vi "Main - ESTF.vi"() -> ()   [LabVIEW 2015]
uses:
  Custom Controls/Main Menu.ctl
  <vilib>/DAQmx/read.llb/DAQmx Read (Analog 1D Wfm NChan NSamp).vi
  <vilib>/DAQmx/miscellaneous.llb/DAQmx Fill In Error Info.vi
  <vilib>/DAQmx/configure/task.llb/DAQmx Configure Logging (TDMS).vi
panel:
  out "Shot complete":bool
  out "Test Permit":bool
  out "HV Enable On?":bool
  in  "stop":bool
  out "HV On Relay":bool
  out "Earthed":bool
  out "Safety System Interlock":bool
  out "Menu":T1
  in  "Max Test Voltage (V)":dbl format="%#_4p"
  in  "Stick Type":string
  in  "Submit Setup":bool
  in  "Test Sequence":T2(array[cluster]) {"Total Test Energy (J)" format="%#_4p"}
  in  "Log File Folderpath":path
  out "Test Information":T3(array[cluster])
  in  "View last Summary":bool
  in  "Unlock Encloure Door":bool
  in  "Back to Setup 2":bool
  in  "Back to Setup":bool
  in  "Data Display":T4(tab)
  out "System Voltage":waveform(dbl)(graph)
  out "Measured Current":waveform(dbl)(graph)
  out "Measured Temperature":waveform(dbl)(graph)
  out "Measured PD Voltage":waveform(dbl)(graph)
  out "Elapsed Time (s)":dbl
  out "Cooldown time":dbl
  out "Pulses":i32
  out "Pulse No.":i32
  in  "Create Report":bool
  in  "Finish":bool
  in  "Show Log file":bool
  out "Total Test Energies":dbl[](array[numeric])
  # "Waiting for HV Enable Switch..."
  # "Waiting for Start Sequence button to be pressed..."
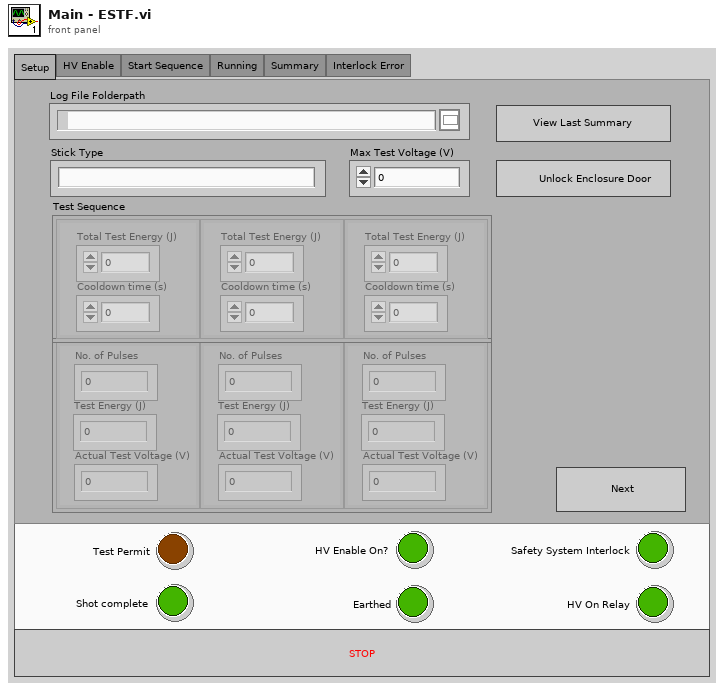
[diagram p1: front panel]
types:
  T1 = typedef "Main Menu.ctl" = enum32{"Setup", "HV Enable", "Start Sequence", "Running", "Summary", "Interlock Error"}
  T2 = cluster{"Cooldown time (s)":dbl, "Total Test Energy (J)":dbl}[]
  T3 = cluster{"No. of Pulses":i32, "Test Energy (J)":dbl, "Actual Test Voltage (V)":dbl}[]
  T4 = enum32{"Voltage", "Current", "Temperature", "PD Voltage"}
  T5 = cluster{"No. of Pulses":i32, "Test Energy (J)":dbl, "Actual Test Voltage (V)":dbl}
  T6 = enum16{"open", "open or create", "create or replace", "create", "open (read-only)"}
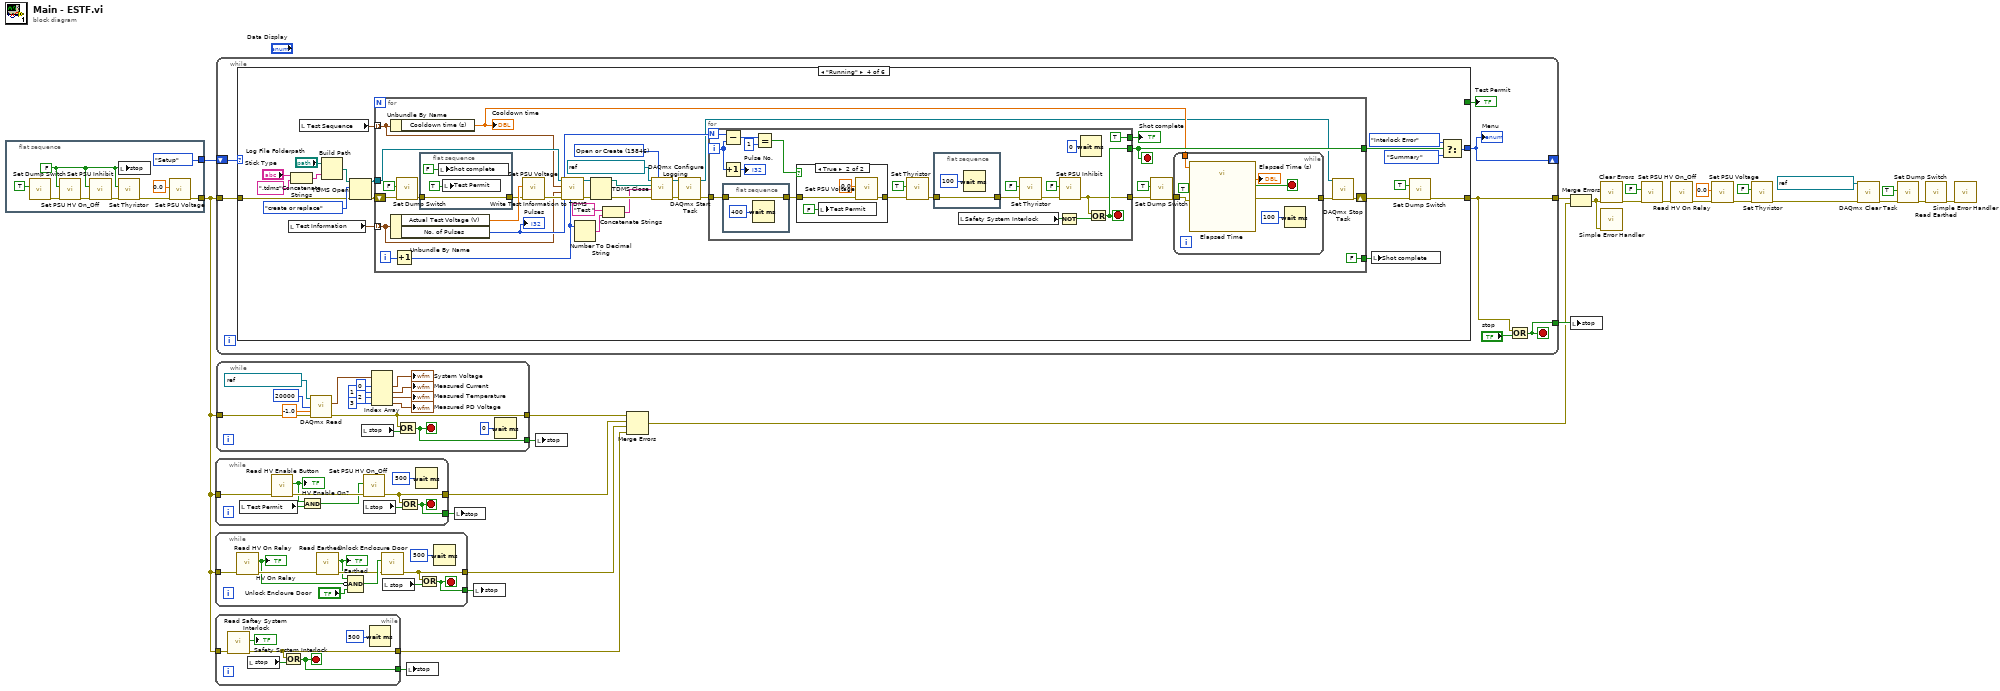
[diagram p0: block diagram]
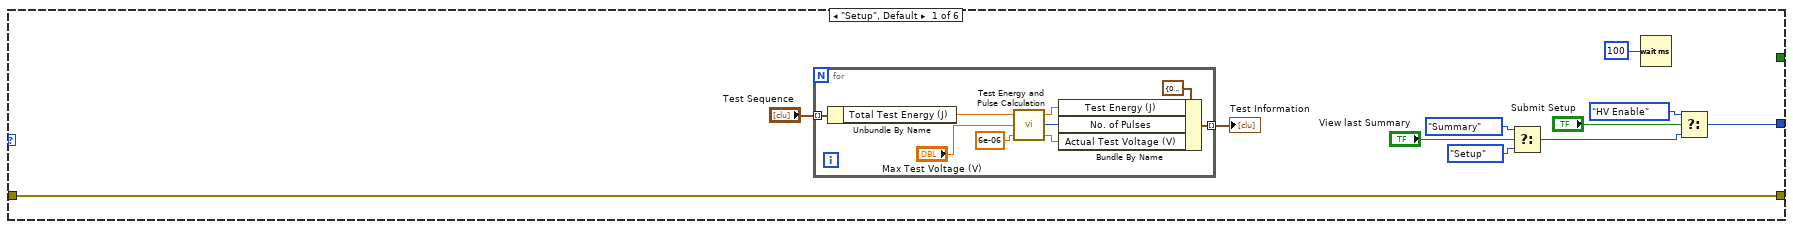
[diagram p2: hidden frame]
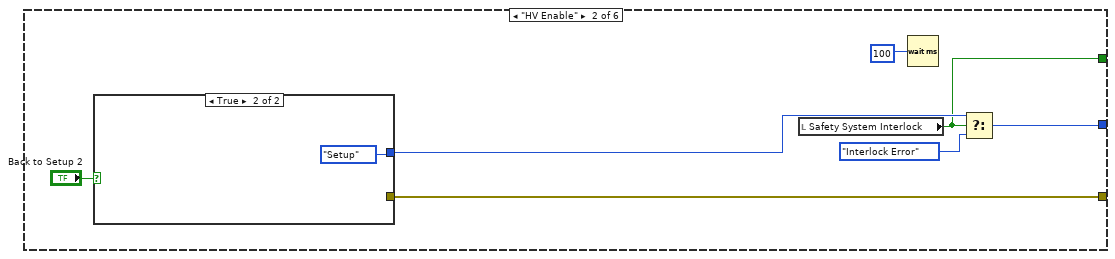
[diagram p3: hidden frame]
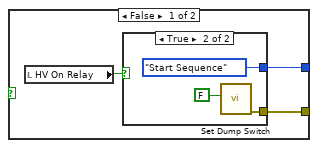
[diagram p4: hidden frame]
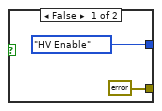
[diagram p5: hidden frame]
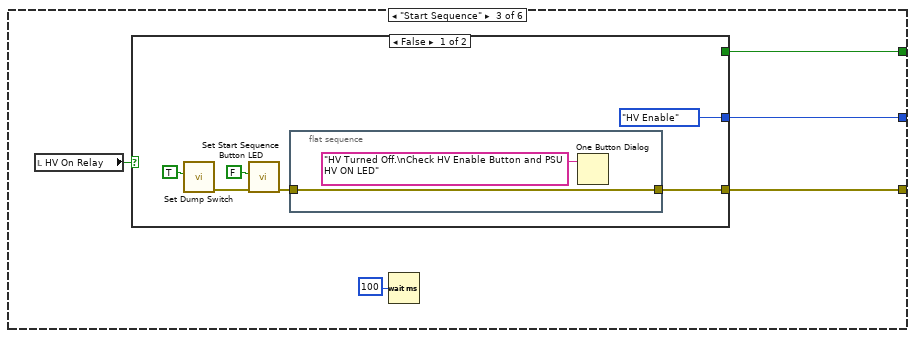
[diagram p6: hidden frame]
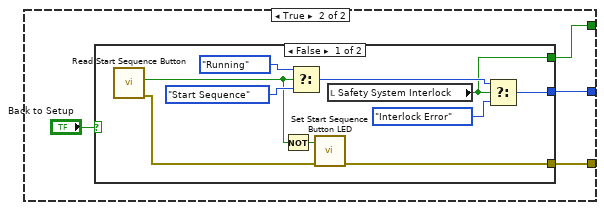
[diagram p7: hidden frame]
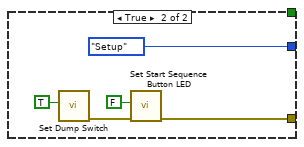
[diagram p8: hidden frame]
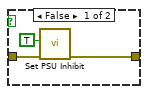
[diagram p9: hidden frame]
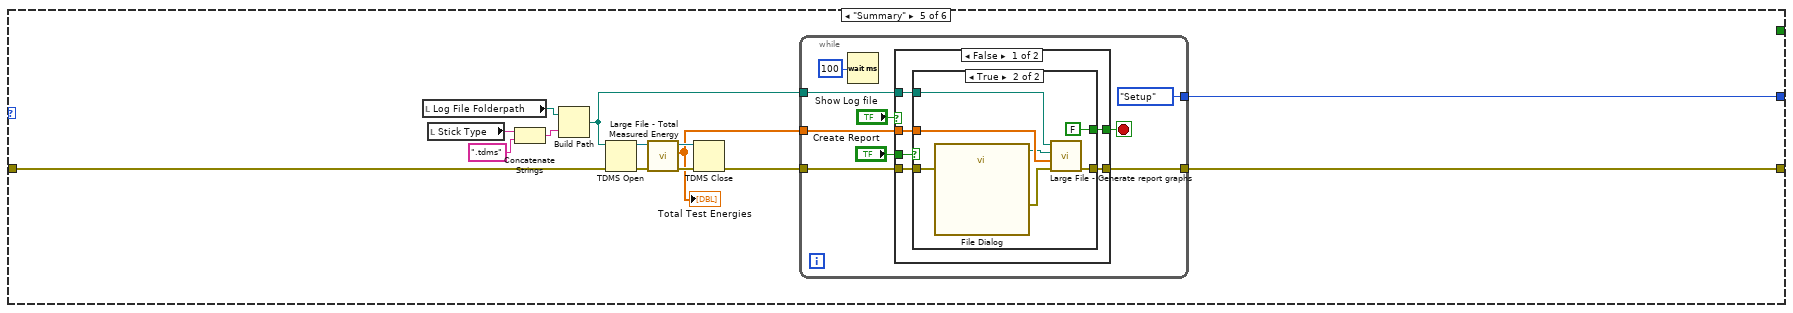
[diagram p10: hidden frame]
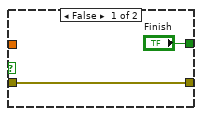
[diagram p11: hidden frame]
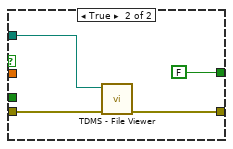
[diagram p12: hidden frame]
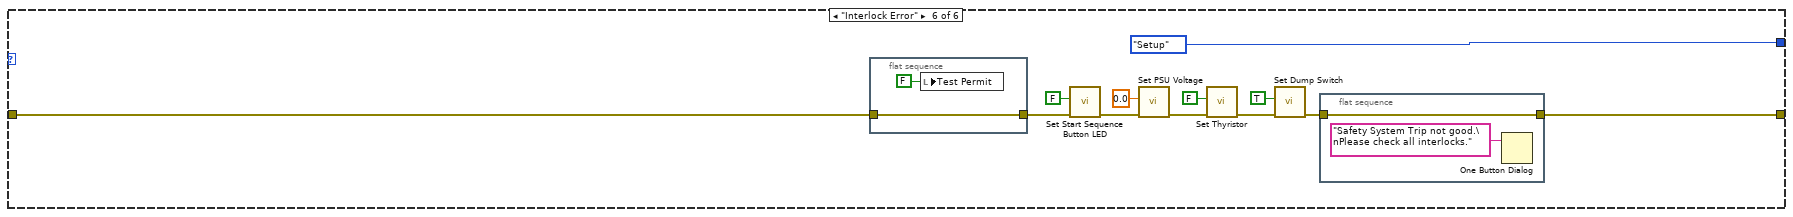
[diagram p13: hidden frame]
diagram:
  n1 = flat-sequence {
    tunnel: [Main_Menu."Setup" ("Menu")] -> w27
    tunnel: [w33] -> w4
    frame #0 {
      w28 = FALSE ("stop")
      n2 = call "Set Dump Switch.vi"("Earth"=TRUE) -> ("error out"=w32:errorcluster)  [unwired: 6 in]
      n3 = call "Set PSU HV On_Off.vi"("error in"=w32, "On/Off"=w28) -> ("error out"=w31:errorcluster)  [unwired: 5 in]
      n4 = call "Set PSU Inhibit.vi"("error in"=w31, "On/Off"=w28) -> ("error out"=w30:errorcluster)  [unwired: 5 in]
      n5 = call "Set Thyristor.vi"("error in"=w30, "On/Off"=w28) -> ("error out"=w29:errorcluster)  [unwired: 5 in]
      n6 = local write "stop"(w28) -> ()
      n7 = call "Set PSU Voltage.vi"("error in"=w29, "Voltage"=0.0) -> ("error out"=w33:errorcluster)  [unwired: 5 in]
    }
  }
  n8 = while {
    tunnel: [w40] -> w10
    tunnel: w4 -> [w39]
    tunnel: [w38] -> w7
    stop <- w40 stop-if-true
    n9 = local read "Test Permit"() -> (w42:bool)
    n10 = call "Read HV Enable Button.vi"("error in"=w39) -> ("error out"=w45:errorcluster, "HV Enable Pressed?"=w43:bool)  [unwired: 5 in]
    "HV Enable On?" <- w43
    n11 = And(x=w43, y=w42) -> (x .and. y?=w44:bool)
    n12 = call "Set PSU HV On_Off.vi"("error in"=w45, "On/Off"=w44) -> ("error out"=w38:errorcluster)  [unwired: 5 in]
    n13 = local read "stop"() -> (w41:bool)
    n14 = Or(x=w38, y=w41) -> (x .or. y?=w40:bool)
    n15 = Wait (ms)(milliseconds to wait=u32 500) -> ()  [unwired: 1 out]
  }
  n16 = while {
    tunnel: [w51] -> w11
    tunnel: w4 -> [w48]
    tunnel: [w47] -> w5
    stop <- w51 stop-if-true
    n17 = call "Read HV On Relay.vi"("error in"=w48) -> ("error out"=w56:errorcluster, "HV On Relay"=w55:bool)  [unwired: 5 in]
    "HV On Relay" <- w55
    n18 = call "Read Earthed.vi"("error in"=w56) -> ("error out"=w53:errorcluster, "Dump Switch mimic"=w50:bool)  [unwired: 5 in]
    "Earthed" <- w50
    n19 = Compound Arithmetic op=AND(w50, invert w55, "Unlock Encloure Door") -> (w54:bool)
    n20 = call "Unlock Enclosure Door.vi"("error in"=w53, "Unlock Encloure Door"=w54) -> ("error out"=w47:errorcluster)  [unwired: 5 in]
    n21 = local read "stop"() -> (w52:bool)
    n22 = Or(x=w47, y=w52) -> (x .or. y?=w51:bool)
    n23 = Wait (ms)(milliseconds to wait=u32 500) -> ()  [unwired: 1 out]
  }
  n24 = while {
    tunnel: [w61] -> w12
    tunnel: w4 -> [w59]
    tunnel: [w58] -> w6
    stop <- w61 stop-if-true
    n25 = call "Read Saftey System Interlock.vi"("error in"=w59) -> ("error out"=w58:errorcluster, "Safety System Interlock"=→"Safety System Interlock":bool)  [unwired: 5 in]
    n26 = local read "stop"() -> (w60:bool)
    n27 = Or(x=w58, y=w60) -> (x .or. y?=w61:bool)
    n28 = Wait (ms)(milliseconds to wait=u32 500) -> ()  [unwired: 1 out]
  }
  n29 = while {
    shift-right: [w66] -> _
    shift-left: w27 -> [w67]
    tunnel: [w68] -> w25
    tunnel: w4 -> [w64]
    tunnel: [w63] -> w1
    stop <- w68 stop-if-true
    n30 = case shown="\"Running\"" w67 {
      tunnel: [w75 w95 w110 w140 w246 Main_Menu."Setup" ("Menu")] -> w66
      tunnel: [w70 w92 w109 w138 w244 w278] -> w63
      tunnel: [_ w91 w108 _ _ _] -> w65
      tunnel: w64 -> [w70 _ _ w144 w243 w275]
      frame "Setup", Default {
        n31 = for {
          tunnel: "Test Sequence" -> [w87] mode=indexing
          tunnel: [w81] -> w78 mode=indexing
          n32 = Unbundle By Name(w87) -> ("Total Test Energy (J)"=w86:dbl)
          n33 = call "Test Energy and Pulse Calculation.vi"("Capacitor Size (f)"=6e-06, "Max Test Voltage (V)"="Max Test Voltage (V)", "Stick Energy (J)"=w86) -> ("Actual Test Voltage (V)"=w82:dbl, "Actual No. of Pulses"=w83:i32, "Actual Pulse Energy (J)"=w84:dbl)
          n34 = Bundle By Name(cluster=T5 {"No. of Pulses"=0, "Test Energy (J)"=0.0, "Actual Test Voltage (V)"=0.0} ("Test Information 2"), "Test Energy (J)"=w84, "No. of Pulses"=w83, "Actual Test Voltage (V)"=w82) -> (w81:T5)
        }
        "Test Information" <- w78
        n35 = Select(t=Main_Menu."Summary" ("Menu"), s="View last Summary", f=Main_Menu."Setup" ("Menu")) -> (s? t:f=w73:T1)
        n36 = Wait (ms)(milliseconds to wait=u32 100) -> ()  [unwired: 1 out]
        n37 = Select(t=Main_Menu."HV Enable" ("Menu"), s="Submit Setup", f=w73) -> (s? t:f=w75:T1)
      }
      frame "HV Enable" {
        n38 = case shown="True" "Back to Setup 2" {
          tunnel: [w99 Main_Menu."Setup" ("Menu")] -> w96
          tunnel: [w98 _] -> w92
          frame False {
            n39 = local read "HV On Relay"() -> (w97:bool)
            n40 = case shown="True" w97 {
              tunnel: [Main_Menu."HV Enable" ("Menu") Main_Menu."Start Sequence" ("Menu")] -> w99
              tunnel: [errorcluster {"status"=FALSE, "code"=0, "source"=""} ("error out") w102] -> w98
              frame False {
              }
              frame True {
                n41 = call "Set Dump Switch.vi"("Earth"=FALSE) -> ("error out"=w102:errorcluster)  [unwired: 6 in]
              }
            }
          }
          frame True {
          }
        }
        n42 = local read "Safety System Interlock"() -> (w91:bool)
        n43 = Wait (ms)(milliseconds to wait=u32 100) -> ()  [unwired: 1 out]
        n44 = Select(t=w96, s=w91, f=Main_Menu."Interlock Error" ("Menu")) -> (s? t:f=w95:T1)
      }
      frame "Start Sequence" {
        n45 = local read "HV On Relay"() -> (w106:bool)
        n46 = case shown="False" w106 {
          tunnel: [Main_Menu."HV Enable" ("Menu") w122] -> w110
          tunnel: [w112 w121] -> w109
          tunnel: [_ w120] -> w108
          frame False {
            n47 = call "Set Dump Switch.vi"("Earth"=TRUE) -> ("error out"=w113:errorcluster)  [unwired: 6 in]
            n48 = call "Set Start Sequence Button LED.vi"("error in"=w113, "Start LED"=FALSE) -> ("error out"=w111:errorcluster)  [unwired: 5 in]
            n49 = flat-sequence {
              tunnel: [w117] -> w112
              tunnel: w111 -> [w117]
              frame #0 {
                n50 = One Button Dialog(message="HV Turned Off.\nCheck HV Enable Button and PSU HV ON LED") -> ()  [unwired: 1 in, 1 out]
              }
            }
          }
          frame True {
            n51 = case shown="False" "Back to Setup" {
              tunnel: [w128 Main_Menu."Setup" ("Menu")] -> w122
              tunnel: [w127 w136] -> w121
              tunnel: [w125 _] -> w120
              frame False {
                n52 = call "Read Start Sequence Button.vi"() -> ("error out"=w123:errorcluster, "Start Button Pressed?"=w124:bool)  [unwired: 6 in]
                n53 = Not(x=w124) -> (.not. x?=w126:bool)
                n54 = Select(t=Main_Menu."Running" ("Menu"), s=w124, f=Main_Menu."Start Sequence" ("Menu")) -> (s? t:f=w129:T1)
                n55 = call "Set Start Sequence Button LED.vi"("error in"=w123, "Start LED"=w126) -> ("error out"=w127:errorcluster)  [unwired: 5 in]
                n56 = local read "Safety System Interlock"() -> (w125:bool)
                n57 = Select(t=w129, s=w125, f=Main_Menu."Interlock Error" ("Menu")) -> (s? t:f=w128:T1)
              }
              frame True {
                n58 = call "Set Dump Switch.vi"("Earth"=TRUE) -> ("error out"=w134:errorcluster)  [unwired: 6 in]
                n59 = call "Set Start Sequence Button LED.vi"("error in"=w134, "Start LED"=FALSE) -> ("error out"=w136:errorcluster)  [unwired: 5 in]
              }
            }
          }
        }
        n60 = Wait (ms)(milliseconds to wait=u32 100) -> ()  [unwired: 1 out]
      }
      frame "Running" {
        n61 = local read "Test Information"() -> (w156:T3)
        n62 = Concatenate Strings("Stick Type", ".tdms" ("string")) -> (w151:string)
        n63 = local read "Test Sequence"() -> (w155:T2)
        n64 = Build Path(base path="Log File Folderpath", name or relative path=w151) -> (appended path=w152:path)
        n65 = TDMS Open(8:w144, 10:T6."create or replace" ("operation (0:open)"), 11:w152) -> (0:w146:errorcluster, 3:w145:refnum<k34>)  [unwired: 4 in]
        n66 = for {
          tunnel: w156 -> [w178] mode=indexing
          tunnel: w155 -> [w179] mode=indexing
          tunnel: w145 -> [w180]
          tunnel: [w182] -> w141
          tunnel: [FALSE] -> w139
          shift-right: [w161] -> w154
          shift-left: w146 -> [w187]
          i -> [w184]
          stop <- w182 stop-if-true
          w169 = 15846 items=["Open"=10437, "Open or Create"=15846, "Create or Replace"=15847, "Create"=15848] ("operation")
          n67 = Unbundle By Name(w178) -> ("Actual Test Voltage (V)"=w189:dbl, "No. of Pulses"=w190:i32)
          "Pulses" <- w190
          n68 = Unbundle By Name(w179) -> ("Cooldown time (s)"=w158:dbl)
          "Cooldown time" <- w158
          n69 = Increment(x=w184) -> (x+1=w168:i32)
          n70 = call "Set Dump Switch.vi"("error in"=w187, "Earth"=FALSE) -> ("error out"=w185:errorcluster)  [unwired: 5 in]
          n71 = flat-sequence {
            tunnel: [w200] -> w186
            tunnel: w185 -> [w200]
            frame #0 {
              n72 = local write "Shot complete"(FALSE ("Shot complete")) -> ()
              n73 = local write "Test Permit"(TRUE ("Test Permit")) -> ()
            }
          }
          n74 = call "Set PSU Voltage.vi"("error in"=w186, "Voltage"=w189) -> ("error out"=w181:errorcluster)  [unwired: 5 in]
          n75 = call "Write Test Information to TDMS.vi"("Test No."=w168, "error in (no error)"=w181, "Test Information"=w178, "Test Sequence"=w179, "Refnum in"=w180) -> ("error out"=w174:errorcluster, "Refnum out"=w173:refnum<k34>)  [unwired: 5 in]
          n76 = Number To Decimal String(number=w168) -> (decimal integer string=w166:string)  [unwired: 1 in]
          n77 = TDMS Close(8:w174, 11:w173) -> (0:w172:errorcluster, 3:w171:path)
          n78 = Concatenate Strings("Test ", w166) -> (w165:string)
          n79 = call-poly <vilib>:"DAQmx Configure Logging.vi"("task/channels in"=refnum<k21> "AI DAQmx Task" ("DAQmx Task Name"), "operation"=w169, "file path"=w171, "group name"=w165, "error in"=w172) -> ("task out"=w162:refnum<k21>, "error out"=w164:errorcluster)  [unwired: 9 in]
          n80 = call <vilib>:"DAQmx Start Task.vi"("task/channels in"=w162, "error in"=w164) -> ("task out"=w157:refnum<k21>, "error out"=w163:errorcluster)  [unwired: 12 in]
          n81 = for {
            N: w190 -> [w221]
            tunnel: w163 -> [w209]
            tunnel: [w203] -> w175
            tunnel: [w204] -> w182
            tunnel: [TRUE] -> w177
            i -> [w212]
            stop <- w204 stop-if-true
            n82 = Subtract(x=w221, y=w212) -> (x-y=w220:i32)
            n83 = Increment(x=w212) -> (x+1=→"Pulse No.":i32)
            n84 = flat-sequence {
              tunnel: [w224] -> w210
              tunnel: w209 -> [w224]
              frame #0 {
                n85 = Wait (ms)(milliseconds to wait=u32 400) -> ()  [unwired: 1 out]
              }
            }
            n86 = Equal?(x=w220, y=1) -> (x = y?=w216:bool)
            n87 = case shown="True" w216 {
              tunnel: w210 -> [w228 w229]
              tunnel: [w226 w232] -> w211
              frame False {
                n88 = call "Set PSU Inhibit.vi"("error in"=w228, "On/Off"=TRUE) -> ("error out"=w226:errorcluster)  [unwired: 5 in]
              }
              frame True {
                n89 = local write "Test Permit"(FALSE ("Test Permit")) -> ()
                n90 = call "Set PSU Voltage.vi"("error in"=w229, "Voltage"=0.0) -> ("error out"=w232:errorcluster)  [unwired: 5 in]
              }
            }
            n91 = call "Set Thyristor.vi"("error in"=w211, "On/Off"=TRUE) -> ("error out"=w208:errorcluster)  [unwired: 5 in]
            n92 = flat-sequence {
              tunnel: [w222] -> w207
              tunnel: w208 -> [w222]
              frame #0 {
                n93 = Wait (ms)(milliseconds to wait=u32 100) -> ()  [unwired: 1 out]
              }
            }
            n94 = local read "Safety System Interlock"() -> (w218:bool)
            n95 = call "Set Thyristor.vi"("error in"=w207, "On/Off"=FALSE) -> ("error out"=w214:errorcluster)  [unwired: 5 in]
            n96 = Not(x=w218) -> (.not. x?=w217:bool)
            n97 = call "Set PSU Inhibit.vi"("error in"=w214, "On/Off"=FALSE) -> ("error out"=w203:errorcluster)  [unwired: 5 in]
            n98 = Wait (ms)(milliseconds to wait=u32 0) -> ()  [unwired: 1 out]
            n99 = Or(x=w203, y=w217) -> (x .or. y?=w204:bool)
          }
          "Shot complete" <- w177
          n100 = call "Set Dump Switch.vi"("error in"=w175, "Earth"=TRUE) -> ("error out"=w160:errorcluster)  [unwired: 5 in]
          n101 = while {
            tunnel: [w194] -> w159
            tunnel: w158 -> [w197]
            tunnel: w160 -> [w192]
            stop <- w195 stop-if-true
            n102 = call "Elapsed Time"("Time Target (s)"=w197, "Auto Reset"=TRUE, "error in (no error)"=w192) -> ("Elapsed Time (s)"=→"Elapsed Time (s)":dbl, "Time has Elapsed"=w195:bool, "error out"=w194:errorcluster)  [unwired: 9 in, 5 out]
            n103 = Wait (ms)(milliseconds to wait=u32 100) -> ()  [unwired: 1 out]
          }
          n104 = call <vilib>:"DAQmx Stop Task.vi"("task/channels in"=w157, "error in"=w159) -> ("error out"=w161:errorcluster)  [unwired: 12 in, 1 out]
        }
        n105 = local write "Shot complete"(w139) -> ()
        n106 = call "Set Dump Switch.vi"("error in"=w154, "Earth"=TRUE) -> ("error out"=w138:errorcluster)  [unwired: 5 in]
        n107 = Select(t=Main_Menu."Interlock Error" ("Menu"), s=w141, f=Main_Menu."Summary" ("Menu")) -> (s? t:f=w140:T1)
      }
      frame "Summary" {
        n108 = local read "Log File Folderpath"() -> (w240:path)
        n109 = local read "Stick Type"() -> (w239:string)
        n110 = Concatenate Strings(w239, ".tdms" ("string")) -> (w242:string)
        n111 = Build Path(base path=w240, name or relative path=w242) -> (appended path=w238:path)
        n112 = TDMS Open(8:w243, 11:w238) -> (0:w237:errorcluster, 3:w236:refnum<k34>)  [unwired: 5 in]
        n113 = call "Large File - Total Measured Energy.vi"("error in"=w237, "tdms file"=w236) -> ("error out"=w234:errorcluster, "Total Test Energies (J)"=w233:dbl[], "tdms file out"=w235:refnum<k34>)  [unwired: 3 in]
        "Total Test Energies" <- w233
        n114 = TDMS Close(8:w234, 11:w235) -> (0:w245:errorcluster)  [unwired: 1 out]
        n115 = while {
          tunnel: w238 -> [w253]
          tunnel: [Main_Menu."Setup" ("Menu")] -> w246
          tunnel: w245 -> [w249]
          tunnel: [w248] -> w244
          tunnel: w233 -> [w247]
          stop <- w255 stop-if-true
          n116 = Wait (ms)(milliseconds to wait=u32 100) -> ()  [unwired: 1 out]
          n117 = case shown="False" "Show Log file" {
            tunnel: [w261 FALSE ("Finish")] -> w255
            tunnel: w253 -> [w257 w273]
            tunnel: "Create Report" -> [w260 _]
            tunnel: w249 -> [w259 w272]
            tunnel: [w258 w271] -> w248
            tunnel: w247 -> [w256 _]
            frame False {
              n118 = case shown="True" w260 {
                tunnel: ["Finish" FALSE ("Finish")] -> w261
                tunnel: w259 -> [w262 w269]
                tunnel: [w262 w267] -> w258
                tunnel: w257 -> [_ w265]
                tunnel: w256 -> [_ w266]
                frame False {
                }
                frame True {
                  n119 = call "File Dialog"("error in"=w269) -> ("selected path"=w264:path, "error out"=w268:errorcluster)  [unwired: 11 in, 2 out]
                  n120 = call "Large File - Generate report graphs.vi"("error in (no error)"=w268, "Test Energies"=w266, "report file path"=w264, "file path"=w265) -> ("error out"=w267:errorcluster)  [unwired: 7 in]
                }
              }
            }
            frame True {
              n121 = call <vilib>:"TDMS - File Viewer.vi"("error in (no error)"=w272, "file path"=w273) -> ("error out"=w271:errorcluster)  [unwired: 4 in, 1 out]
            }
          }
        }
      }
      frame "Interlock Error" {
        n122 = flat-sequence {
          tunnel: [w287] -> w277
          tunnel: w275 -> [w287]
          frame #0 {
            n123 = local write "Test Permit"(FALSE ("Test Permit")) -> ()
          }
        }
        n124 = call "Set Start Sequence Button LED.vi"("error in"=w277, "Start LED"=FALSE) -> ("error out"=w276:errorcluster)  [unwired: 5 in]
        n125 = call "Set PSU Voltage.vi"("error in"=w276, "Voltage"=0.0 ("data")) -> ("error out"=w282:errorcluster)  [unwired: 5 in]
        n126 = call "Set Thyristor.vi"("error in"=w282, "On/Off"=FALSE ("data")) -> ("error out"=w281:errorcluster)  [unwired: 5 in]
        n127 = call "Set Dump Switch.vi"("error in"=w281, "Earth"=TRUE) -> ("error out"=w279:errorcluster)  [unwired: 5 in]
        n128 = flat-sequence {
          tunnel: [w289] -> w278
          tunnel: w279 -> [w289]
          frame #0 {
            n129 = One Button Dialog(message="Safety System Trip not good.\nPlease check all interlocks.") -> ()  [unwired: 1 in, 1 out]
          }
        }
      }
    }
    "Menu" <- w66
    "Test Permit" <- w65
    n130 = Or(x=w63, y="stop") -> (x .or. y?=w68:bool)
  }
  n131 = while {
    tunnel: w4 -> [w307]
    tunnel: [w292] -> w3
    tunnel: [w293] -> w2
    stop <- w293 stop-if-true
    n132 = call-poly <vilib>:"DAQmx Read.vi"("task/channels in"=refnum<k21> "AI DAQmx Task" ("DAQmx Task Name"), "number of samples per channel"=20000, "timeout"=-1.0, "error in"=w307) -> ("data"=w295:waveform(dbl)[], "error out"=w292:errorcluster)  [unwired: 9 in, 1 out]
    n133 = local read "stop"() -> (w294:bool)
    n134 = Index Array(array=w295, index #1=0 ("index"), index #2=1 ("index"), index #3=2 ("index"), index #4=3 ("index")) -> (element #1=→"System Voltage":waveform(dbl), element #2=→"Measured Current":waveform(dbl), element #3=→"Measured Temperature":waveform(dbl), element #4=→"Measured PD Voltage":waveform(dbl))
    n135 = Or(x=w292, y=w294) -> (x .or. y?=w293:bool)
    n136 = Wait (ms)(milliseconds to wait=u32 0) -> ()  [unwired: 1 out]
  }
  n137 = local write "stop"(w12) -> ()
  n138 = local write "stop"(w10) -> ()
  n139 = local write "stop"(w11) -> ()
  n140 = local write "stop"(w2) -> ()
  n141 = Merge Errors(w3, w7, w5, w6) -> (w9:errorcluster)
  n142 = Merge Errors(w1, w9) -> (w21:errorcluster)
  n143 = local write "stop"(w25) -> ()
  n144 = call <vilib>:"Clear Errors.vi"("error in (no error)"=w21) -> ("error out"=w19:errorcluster)  [unwired: 5 in, 1 out]
  n145 = call <vilib>:"Simple Error Handler.vi"("error in (no error)"=w21) -> ()  [unwired: 4 in, 5 out]
  n146 = call "Set PSU HV On_Off.vi"("error in"=w19, "On/Off"=FALSE ("data")) -> ("error out"=w14:errorcluster)  [unwired: 5 in]
  n147 = call "Read HV On Relay.vi"("error in"=w14) -> ("error out"=w13:errorcluster)  [unwired: 5 in, 1 out]
  n148 = call "Set PSU Voltage.vi"("error in"=w13, "Voltage"=0.0 ("data")) -> ("error out"=w17:errorcluster)  [unwired: 5 in]
  n149 = call "Set Thyristor.vi"("error in"=w17, "On/Off"=FALSE ("data")) -> ("error out"=w15:errorcluster)  [unwired: 5 in]
  n150 = call <vilib>:"DAQmx Clear Task.vi"("task in"=refnum<k21> "AI DAQmx Task" ("DAQmx Task Name"), "error in"=w15) -> ("error out"=w23:errorcluster)  [unwired: 13 in]
  n151 = call "Set Dump Switch.vi"("error in"=w23, "Earth"=TRUE) -> ("error out"=w22:errorcluster)  [unwired: 5 in]
  n152 = call "Read Earthed.vi"("error in"=w22) -> ("error out"=w8:errorcluster)  [unwired: 5 in, 1 out]
  n153 = call <vilib>:"Simple Error Handler.vi"("error in (no error)"=w8) -> ()  [unwired: 4 in, 5 out]
